vi "Read hostname.vi"(11 "address":refnum<class "Hostname Network Address.lvclass">) -> (2 "hostname":string, 3 "address out":refnum<class "Hostname Network Address.lvclass">)   [LabVIEW 2020, in "NI_WFCN.lvlib" / "Hostname Network Address.lvclass"]
doc: "Return the hostname this object encapsulates."
uses:
  <vilib>/net/WFCN/Addressing/Hostname Network Address/Hostname Network Address.lvclass
  <vilib>/net/WFCN/Addressing/Hostname Network Address/Hostname Network Address.lvclass/Hostname Network Address.ctl
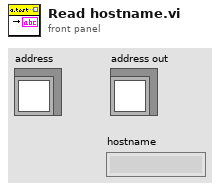
[diagram p1: front panel]
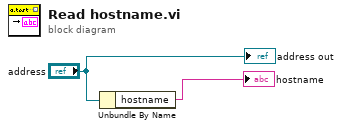
[diagram p0: block diagram]
diagram:
  n1 = Unbundle By Name("address") -> ("hostname"=→"hostname":string)
  "address out" <- "address"
